vi "prac1-2.vi"(0 "Grados Farenheit":dbl) -> (1 "Grados Celcius":dbl(slide) scale=0.0..100.0, 2 "Grados Rankine":dbl(slide) scale=0.0..1000.0, 3 "Grados Kelvin":dbl(slide) scale=0.0..1000.0)   [LabVIEW 2014]
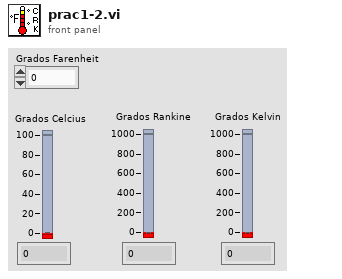
[diagram p1: front panel]
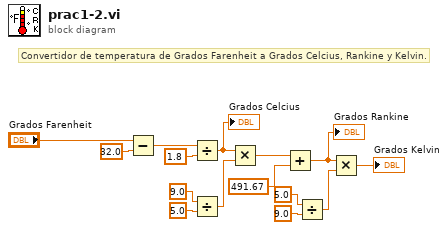
[diagram p0: block diagram]
diagram:
  # "Convertidor de temperatura de Grados Farenheit a Grados Celcius, Rankine y Kelvin."
  n1 = Subtract(x="Grados Farenheit", y=32.0) -> (x-y=w14:dbl)
  n2 = Divide(x=w14, y=1.8) -> (x/y=w8:dbl)
  "Grados Celcius" <- w8
  n3 = Divide(x=9.0, y=5.0) -> (x/y=w9:dbl)
  n4 = Multiply(x=w8, y=w9) -> (x*y=w7:dbl)
  n5 = Add(x=w7, y=491.67) -> (x+y=w2:dbl)
  "Grados Rankine" <- w2
  n6 = Divide(x=5.0, y=9.0) -> (x/y=w3:dbl)
  n7 = Multiply(x=w2, y=w3) -> (x*y=→"Grados Kelvin":dbl)
